vi "dfd_Complex Number to XY Plot.vi"(10 "upper half plane only":bool, 11 "complex numbers":cdb[](array[numeric])) -> (3 "XY plot":cluster{dbl[], dbl[]})   [LabVIEW 2017, in "NI_DigFilterLicensed.lvlib"]
uses:
  <vilib>/addons/Digital Filter Design/NI_DigFilterLicensed.lvlib
  <vilib>/Analysis/NI_AALPro.lvlib
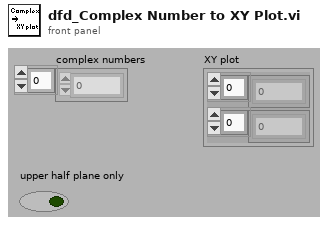
[diagram p1: front panel]
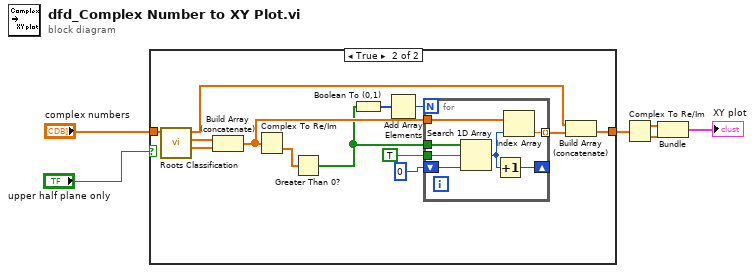
[diagram p0: block diagram]
diagram:
  n1 = case shown="True" "upper half plane only" {
    tunnel: [w7 w20] -> w5
    tunnel: "complex numbers" -> [w7 w8]
    frame False {
    }
    frame True {
      n2 = call <vilib>:"Roots Classification.vi"("Roots"=w8) -> ("Pure Complex Roots"=w10:cdb[], "Complex Pair Roots"=w9:cdb[], "Real Roots"=w19:dbl[])  [unwired: 2 in, 6 out]
      n3 = Build Array (concatenate)(w9, w10) -> (w17:cdb[])
      n4 = Complex To Re/Im(x + iy=w17) -> (y=w11:dbl[])  [unwired: 1 out]
      n5 = Greater Than 0?(x=w11) -> (x > 0?=w15:bool[])
      n6 = Boolean To (0,1)(Boolean=w15) -> (0, 1=w12:i16[])
      n7 = Add Array Elements(numeric array=w12) -> (sum=w13:i16)
      n8 = for {
        N: w13 -> [_]
        shift-right: [w24] -> _
        shift-left: 0 -> [w25]
        tunnel: w15 -> [w27]
        tunnel: TRUE ("element") -> [w26]
        tunnel: w17 -> [w22]
        tunnel: [w21] -> w18 mode=indexing
        n9 = Search 1D Array(1D array=w27, element=w26, start index (0)=w25) -> (index of element=w23:i32)
        n10 = Increment(x=w23) -> (x+1=w24:i32)
        n11 = Index Array(array=w22, index=w23) -> (element=w21:cdb)
      }
      n12 = Build Array (concatenate)(w19, w18) -> (w20:cdb[])
    }
  }
  n13 = Complex To Re/Im(x + iy=w5) -> (x=w3:dbl[], y=w2:dbl[])
  n14 = Bundle(w3, w2) -> (→"XY plot":cluster{dbl[], dbl[]})  [unwired: 1 out]
